vi "LabVIEW PID Controller.vi"(1 "PID Parameters":cluster{"Kp":dbl, "Ti [s]":dbl, "Td [sec]":dbl}={"Kp"=0.5, "Ti [s]"=10.0, "Td [sec]"=0.0}, 2 "Setpoint":dbl=25.0, 3 "Process Variable":dbl) -> (0 "Control Value":dbl)   [LabVIEW 2017]
uses:
  <vilib>/addons/control/pid/pid.llb/PID Advanced (DBL).vi
  <vilib>/addons/control/pid/NI_PID_pid.lvlib
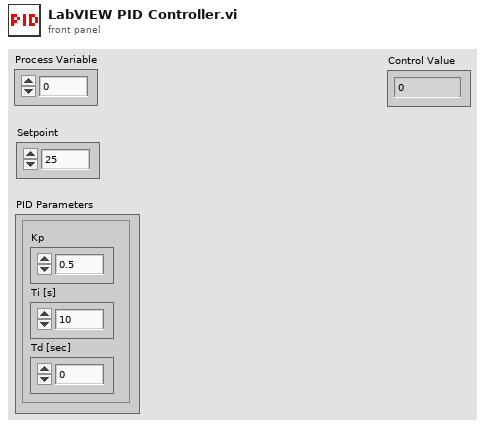
[diagram p1: front panel]
types:
  T1 = cluster{"Kc Scaling":i32, "Ti Scaling":i32, "Td Scaling":i32}
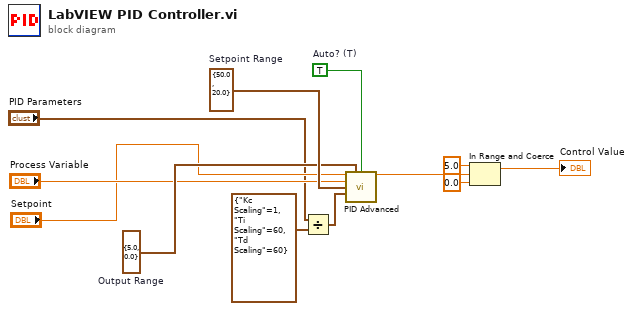
[diagram p0: block diagram]
diagram:
  w12 = TRUE  # Auto? (T)
  w5 = cluster{"output high":dbl, "output low":dbl} {"output high"=5.0, "output low"=0.0}  # Output Range
  w9 = cluster{"Setpoint high":dbl, "Setpoint low":dbl} {"Setpoint high"=50.0, "Setpoint low"=20.0}  # Setpoint Range
  n1 = Divide(x="PID Parameters", y=T1 {"Kc Scaling"=1, "Ti Scaling"=60, "Td Scaling"=60} ("PID Param Scaling")) -> (x/y=w10:cluster{dbl, dbl, dbl})
  n2 = call-poly <vilib>:"PID Advanced.vi"("setpoint"="Setpoint", "output range"=w5, "auto? (T)"=w12, "process variable"="Process Variable", "setpoint range"=w9, "PID gains"=w10) -> ("output"=w6:dbl)  [unwired: 8 in, 1 out]
  n3 = In Range and Coerce(upper limit=5.0, x=w6, lower limit=0.0) -> (coerced(x)=→"Control Value":dbl)  [unwired: 1 out]
